vi "mqttWillReadvi.vi"(8 "error in (no error)":errorcluster, 11 "mqtt in":refnum<class "mqtt.lvclass">) -> (0 "error out":errorcluster, 2 "Will Info":T1={"Will message"="Last Will", "Will Topic"="Will Topic"}, 3 "mqtt out":refnum<class "mqtt.lvclass">)   [LabVIEW 2015, in "mqtt.lvclass"]
uses:
  mqtt.lvclass
  mqttTypedef/mqttUserInformation.ctl
  mqtt.lvclass/mqtt.ctl
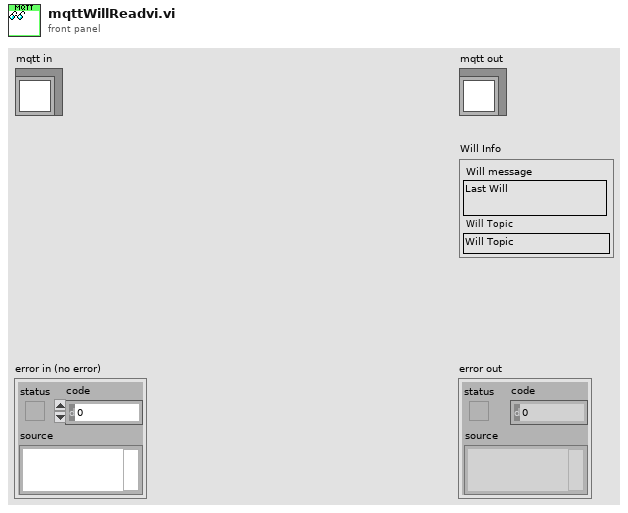
[diagram p1: front panel]
types:
  T1 = typedef "mqttUserInformation.ctl" = cluster{"Will message":string, "Will Topic":string}
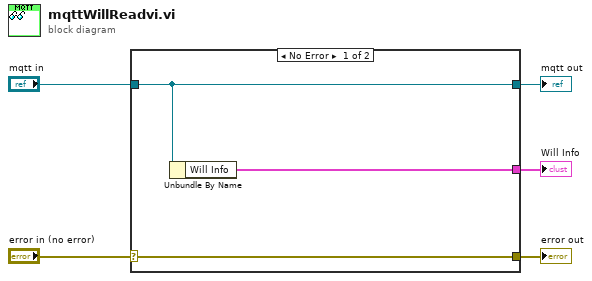
[diagram p0: block diagram]
diagram:
  n1 = case shown="No Error" "error in (no error)" {
    selector: "error in (no error)" -> [w8 w9]
    tunnel: [w8 w9] -> w4
    tunnel: [w7 w10] -> w2
    tunnel: "mqtt in" -> [w7 w10]
    tunnel: [w6 _] -> w1
    frame No Error {
      n2 = Unbundle By Name(w7) -> ("Will Info"=w6:T1)
    }
    frame Error {
    }
  }
  "error out" <- w4
  "mqtt out" <- w2
  "Will Info" <- w1
